vi "setUp.vi"(8 "error in (no error)":errorcluster, 11 "reference in":refnum<class "Add User.lvclass">) -> (0 "error out":errorcluster, 3 "reference out":refnum<class "Add User.lvclass">)   [LabVIEW 2017, in "Add User.lvclass"]
doc: "setUp runs prior to the test method during test execution. Use this method to initialize any object data required by your tests."
uses:
  Add User.lvclass
  C:/Program Files (x86)/National Instruments/LabVIEW 2017/vi.lib/addons/_JKI Toolkits/VI Tester/TestCase.llb/TestCase.lvclass
  Source/User Configuration Manager/User Configuration Manager.lvclass
  C:/CS Dev/LabVIEW Modules/composed-user-manager/Source/iUser Configuration Manager/iUser Configuration Manager.lvclass
  Add User.lvclass/Add User.ctl
  <vilib>/addons/_JKI Toolkits/VI Tester/TestCase.llb/TestCase.lvclass
  Source/User Configuration Manager Ref/By Ref.lvlib
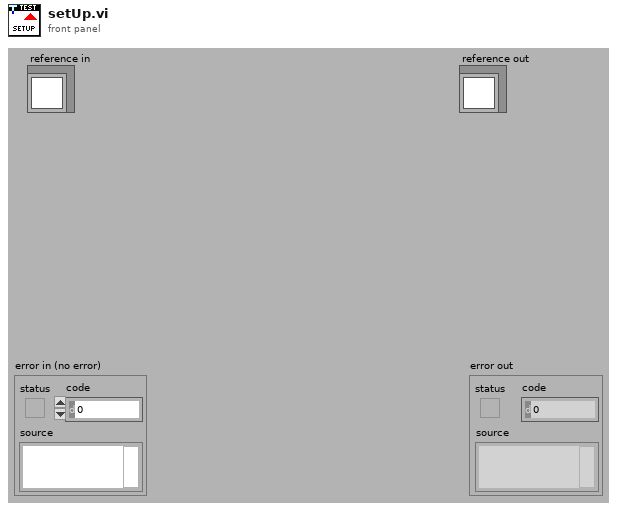
[diagram p1: front panel]
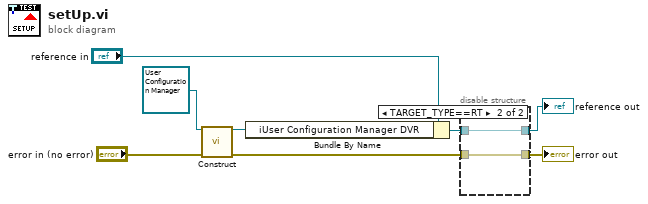
[diagram p0: block diagram]
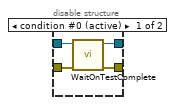
[diagram p2: hidden frame]
diagram:
  n1 = call "Construct.vi"("iUser Configuration Manager in"=refnum<class "User Configuration Manager.lvclass"> refnum ("User Configuration Manager.lvlib:User Configuration Manager"), "error in"="error in (no error)") -> ("dup iUser Configuration Manager DVR"=w3:refnum<data-value>, "error out"=w1:errorcluster)  [unwired: 12 in]
  n2 = Bundle By Name(cluster="reference in", "iUser Configuration Manager DVR"=w3) -> (w5:refnum<class "Add User.lvclass">)
  n3 = disable-structure shown="TARGET_TYPE==RT" {
    disable-tunnel: w1 -> [w12 w13]
    disable-tunnel: [w11 w13] -> w8
    disable-tunnel: [w10 w14] -> w6
    disable-tunnel: w5 -> [w9 w14]
    frame condition #0 (active) {
      n4 = call <vilib>:"WaitOnTestComplete.vi"("error in (no error)"=w12, "TestCase in"=w9) -> ("error out"=w11:errorcluster, "TestCase out"=w10:refnum<class "Add User.lvclass">)  [unwired: 8 in]
    }
    frame condition #1 {
    }
  }
  "error out" <- w8
  "reference out" <- w6
